vi "4155C Output v2.0.vi"(0 "VISA resource name in":refnum<visa-resource-name>="GPIB0::14::INSTR", 1 "Source/Common":u32(ring) items=["SMU1  ", "SMU2  ", "SMU3  ", "SMU4  ", "SMU5  ", "SMU6  "], 2 "Gate":T5={"Gate Start"=0.0, "Gate Stop"=0.0, "Gate Step"=0.0, "Gate Compliance"=0.1, "Gate PComp"=0.0, "Range mode"=0, "Range"=6} {"Range" max=11 scale=0.0..11.0; "Range mode" items=["Auto", "Limited", "Fixed"]; "Gate PComp" format="%^.2e"; "Gate Compliance" format="%^.2e"; "Gate Step" format="%^.4e"; "Gate Stop" format="%^.4e"; "Gate Start" format="%^.4e"}, 3 "Drain":T6={"Drain Start"=0.0, "Drain Stop"=0.0, "Drain Compliance"=0.1, "Drain Step (linear only)"=0.0, "Drain PComp"=0.0, "Range mode"=0, "Range"=6} {"Range" max=11 scale=0.0..11.0; "Range mode" items=["Auto", "Limited", "Fixed"]; "Drain PComp" format="%^.2e"; "Drain Step (linear only)" format="%^.4e"; "Drain Compliance" format="%^.2e"; "Drain Stop" format="%^.4e"; "Drain Start" format="%^.4e"}, 4 "Drain":u32(ring)=1 items=["SMU1  ", "SMU2  ", "SMU3  ", "SMU4  ", "SMU5  ", "SMU6  "], 5 "Timings":T4={"integration time"=0, "Short/Long integration time"=0.00064, "hold time (sec)"=0.0, "delay time (sec)"=0.0, "Step Time (0 disables)"=0.0, "sweep method"=0, "Pulse period"=0.005, "Base voltage"=0.0, "Pulse width"=0.0005} {"Pulse width" min=0.0005 max=0.1 step=0.0001 format="%.4f"; "Base voltage" format="%^.4e"; "Pulse period" min=0.005 max=1.0 step=0.0001 format="%.4f"; "sweep method" items=["Continuous", "Pulsed"]; "Step Time (0 disables)" format="%.2f"; "delay time (sec)" format="%.4f"; "hold time (sec)" format="%.4f"; "Short/Long integration time" format="%^.0e"; "integration time" scale=0.0..2.0}, 6 "error in (no error)":errorcluster, 7 "Probe 4":cluster{"on/off":bool, "Voltage":dbl} {"Voltage" min=-100.0 max=100.0 format="%.2f"}, 8 "Gate":u32(ring)=2 items=["SMU1  ", "SMU2  ", "SMU3  ", "SMU4  ", "SMU5  ", "SMU6  "], 9 "Probe 4":u32(ring)=3 items=["SMU1  ", "SMU2  ", "SMU3  ", "SMU4  ", "SMU5  ", "SMU6  "], 10 "sweep mode":u16(ring) items=["Single", "Double"], 12 "Panel controls":T3={"Emergency Stop"=refnum, "OutputGraph Max"=1e-05, "Text/Graph (text=false)"=FALSE} {"OutputGraph Max" format="%.2e"}, 13 "Standby":T1) -> (16 "VD":dbl[](array[numeric]) format="%.2f", 17 "Outparams":T2={"V2 Start"=0.0, "V2 Step"=0.0, "Number of points"=1} {"V2 Step" format="%.2f"; "V2 Start" format="%^.4e"}, 20 "VISA Resource Name out":refnum<visa-resource-name>, 22 "IS":dbl[](array[numeric]) format="%.2f", 23 "ID":dbl[](array[numeric]) format="%.2f", 25 "IG":dbl[](array[numeric]) format="%.2f", 26 "error out":errorcluster, 27 "Probe 4":dbl[](array[numeric]) format="%.2f")   [LabVIEW 2016]
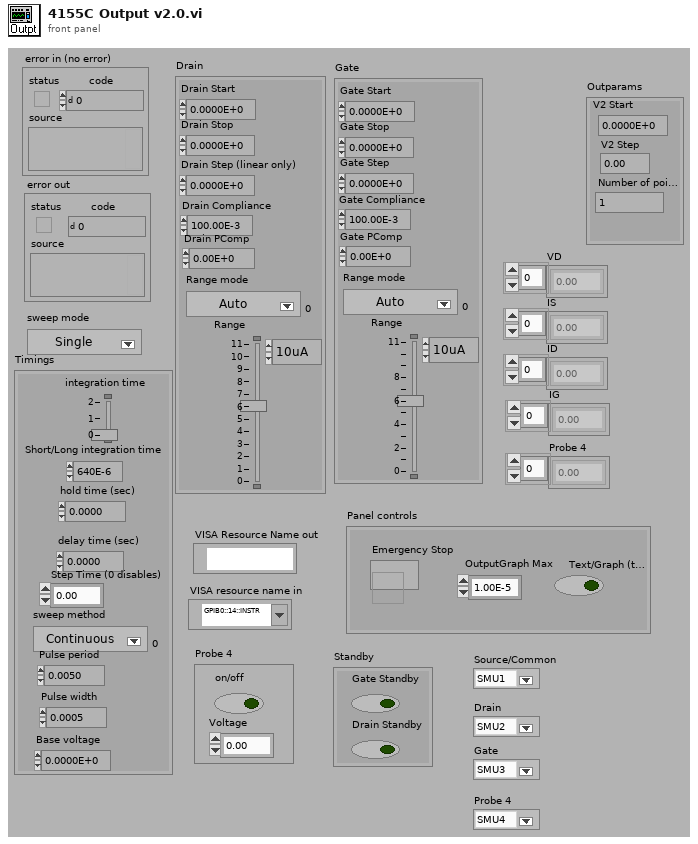
[diagram p1: front panel]
types:
  T1 = cluster{"Gate Standby":bool, "Drain Standby":bool}
  T2 = cluster{"V2 Start":dbl, "V2 Step":dbl, "Number of points":i32}
  T3 = cluster{"Emergency Stop":refnum<vi>, "OutputGraph Max":dbl, "Text/Graph (text=false)":bool}
  T4 = cluster{"integration time":u32, "Short/Long integration time":dbl, "hold time (sec)":dbl, "delay time (sec)":dbl, "Step Time (0 disables)":dbl, "sweep method":u16, "Pulse period":dbl, "Base voltage":dbl, "Pulse width":dbl}
  T5 = cluster{"Gate Start":dbl, "Gate Stop":dbl, "Gate Step":dbl, "Gate Compliance":dbl, "Gate PComp":dbl, "Range mode":u16, "Range":u8}
  T6 = cluster{"Drain Start":dbl, "Drain Stop":dbl, "Drain Compliance":dbl, "Drain Step (linear only)":dbl, "Drain PComp":dbl, "Range mode":u16, "Range":u8}
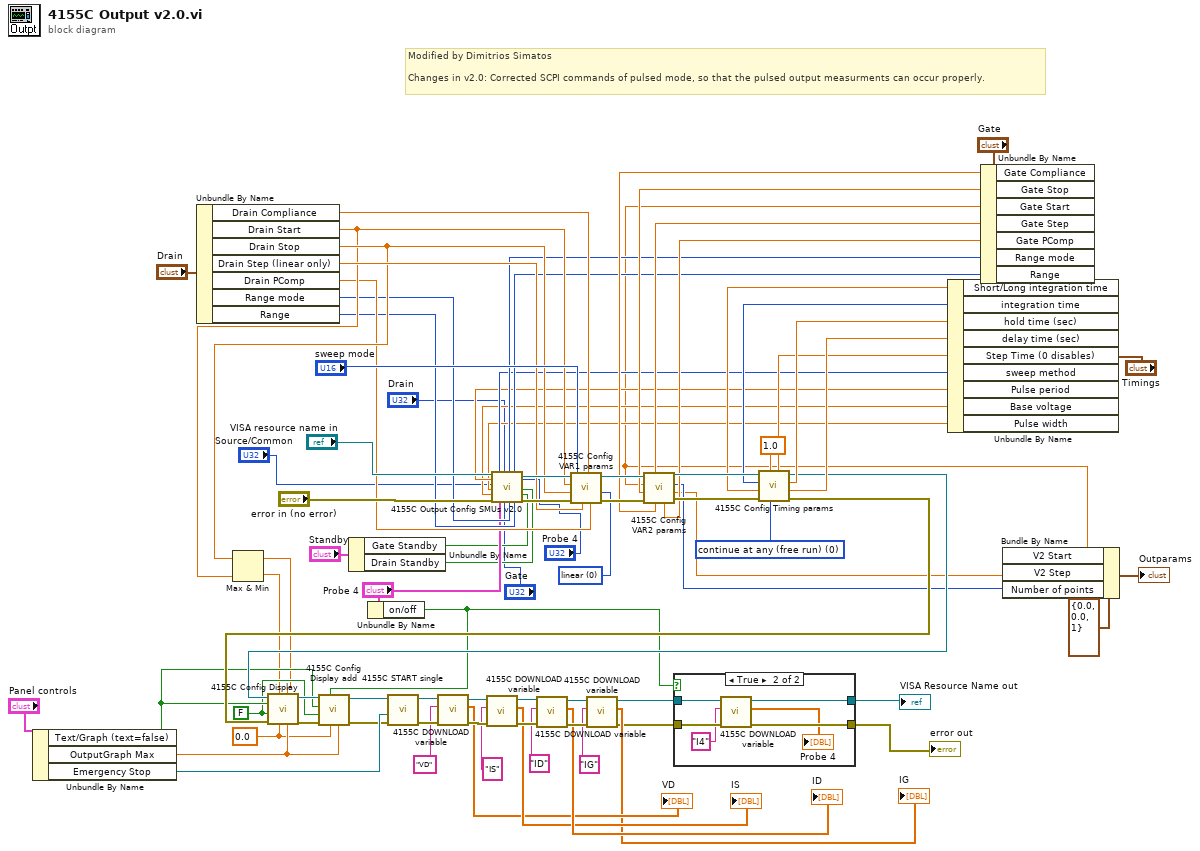
[diagram p0: block diagram]
diagram:
  w8 = 0.0 ("Ymin")
  w9 = FALSE ("Logarithmic")
  w69 = u8 0 items=["continue at any (free run)", "stop at any abnorm", "stop at compliance"] ("stop condition (free run:0)")
  w66 = u16 0 items=["linear", "log 10", "log 25", "log 50"] ("sweep spacing (linear: 0)")
  # "Modified by Dimitrios Simatos\n\nChanges in v2.0: Corrected SCPI commands of pulsed mode, so that the pulsed output measurments can occur properly."
  n1 = Unbundle By Name("Panel controls") -> ("Text/Graph (text=false)"=w10:bool, "OutputGraph Max"=w11:dbl, "Emergency Stop"=w39:refnum<vi>)
  n2 = Unbundle By Name("Drain") -> ("Drain Compliance"=w53:dbl, "Drain Start"=w41:dbl, "Drain Stop"=w42:dbl, "Drain Step (linear only)"=w52:dbl, "Drain PComp"=w38:dbl, "Range mode"=w34:u16, "Range"=w33:u8)
  n3 = Max & Min(x=w42, y=w41) -> (max(x,y)=w6:dbl, min(x,y)=w7:dbl)
  n4 = Unbundle By Name("Standby") -> ("Gate Standby"=w16:bool, "Drain Standby"=w17:bool)
  n5 = Unbundle By Name("Probe 4") -> ("on/off"=w5:bool)
  n6 = Unbundle By Name("Timings") -> ("Short/Long integration time"=w71:dbl, "integration time"=w48:u32, "hold time (sec)"=w49:dbl, "delay time (sec)"=w50:dbl, "Step Time (0 disables)"=w45:dbl, "sweep method"=w32:u16, "Pulse period"=w31:dbl, "Base voltage"=w29:dbl, "Pulse width"=w30:dbl)
  n7 = Unbundle By Name("Gate") -> ("Gate Compliance"=w56:dbl, "Gate Stop"=w55:dbl, "Gate Start"=w24:dbl, "Gate Step"=w54:dbl, "Gate PComp"=w37:dbl, "Range mode"=w36:u16, "Range"=w35:u8)
  n8 = call "4155C Output Config SMUs v2.0.vi"("VISA resource name in"="VISA resource name in", "Pulse period"=w31, "Source/Common"="Source/Common", "Pulse width"=w30, "Base voltage"=w29, "error in (no error)"="error in (no error)", "sweep method"=w32, "SMU4"="Probe 4", "Drain"="Drain", "Gate"="Gate", "Gate mode"=w36, "Source/drain mode"=w34, "Gate Range"=w35, "Source/drain Range"=w33, "Probe 4"="Probe 4", "Drain Standby"=w17, "Gate Standby"=w16) -> ("VISA Resource Name out"=w64:refnum<visa-resource-name>, "error out"=w63:errorcluster)  [unwired: 1 in]
  n9 = call "4155C Config VAR1 params.vi"("sweep spacing (linear: 0)"=w66, "power compliance (0 = OFF)"=w38, "compliance"=w53, "step (linear only)"=w52, "sweep mode"="sweep mode", "error in (no error)"=w63, "stop"=w42, "start"=w41, "VISA session"=w64) -> ("error out"=w67:errorcluster, "dup VISA resource name"=w68:refnum<visa-resource-name>)  [unwired: 1 out]
  n10 = call "4155C Config VAR2 params.vi"("power compliance (0 = OFF)"=w37, "compliance"=w56, "step"=w54, "error in (no error)"=w67, "stop"=w55, "start"=w24, "VISA session"=w68) -> ("error out"=w72:errorcluster, "Corrected Step"=w25:dbl, "Number of points"=w26:i32, "dup VISA resource name"=w73:refnum<visa-resource-name>)  [unwired: 1 in]
  n11 = call "4155C Config Timing params.vi"("delay time (sec)"=w50, "hold time (sec)"=w49, "Step Time (0 disables)"=w45, "stop condition (free run:0)"=w69, "wait time parameter"=1.0, "error in (no error)"=w72, "Short/Long integration time"=w71, "integration time"=w48, "VISA session"=w73) -> ("error out"=w44:errorcluster, "dup VISA resource name"=w43:refnum<visa-resource-name>)  [unwired: 1 in]
  n12 = call "4155C Config Display.vi"("Ymax"=w11, "Var1 Stop"=w6, "Ymin"=w8, "Var1 Start"=w7, "error in (no error)"=w44, "Logarithmic"=w9, "SPA Display"=w10, "VISA session"=w43) -> ("error out"=w12:errorcluster, "dup VISA resource name"=w15:refnum<visa-resource-name>)  [unwired: 2 in]
  n13 = call "4155C Config Display add.vi"("Ymax"=w11, "Ymin"=w8, "SMU4"=w5, "error in (no error)"=w12, "Logarithmic"=w9, "SPA Display"=w10, "VISA session"=w15) -> ("error out"=w13:errorcluster, "dup VISA resource name"=w14:refnum<visa-resource-name>)  [unwired: 3 in]
  n14 = call "4155C START single.vi"("error in (no error)"=w13, "Emergency Stop"=w39, "VISA resource name in"=w14) -> ("error out"=w84:errorcluster, "VISA Resource Name out"=w85:refnum<visa-resource-name>)  [unwired: 3 in]
  n15 = call "4155C DOWNLOAD variable.vi"("error in (no error)"=w84, "Variable name"="VD", "VISA resource name in"=w85) -> ("error out"=w82:errorcluster, "Output data"=→"VD":dbl[], "VISA Resource Name out"=w81:refnum<visa-resource-name>)  [unwired: 2 in]
  n16 = call "4155C DOWNLOAD variable.vi"("error in (no error)"=w82, "Variable name"="IS", "VISA resource name in"=w81) -> ("error out"=w78:errorcluster, "Output data"=→"IS":dbl[], "VISA Resource Name out"=w79:refnum<visa-resource-name>)  [unwired: 2 in]
  n17 = call "4155C DOWNLOAD variable.vi"("error in (no error)"=w78, "Variable name"="ID", "VISA resource name in"=w79) -> ("error out"=w77:errorcluster, "Output data"=→"ID":dbl[], "VISA Resource Name out"=w76:refnum<visa-resource-name>)  [unwired: 2 in]
  n18 = call "4155C DOWNLOAD variable.vi"("error in (no error)"=w77, "Variable name"="IG", "VISA resource name in"=w76) -> ("error out"=w19:errorcluster, "Output data"=→"IG":dbl[], "VISA Resource Name out"=w22:refnum<visa-resource-name>)  [unwired: 2 in]
  n19 = case shown="True" w5 {
    tunnel: w22 -> [w87 w93]
    tunnel: [w87 w90] -> w21
    tunnel: [w86 w91] -> w20
    tunnel: w19 -> [w86 w92]
    frame False {
    }
    frame True {
      n20 = call "4155C DOWNLOAD variable.vi"("error in (no error)"=w92, "Variable name"="I4", "VISA resource name in"=w93) -> ("error out"=w91:errorcluster, "Output data"=→"Probe 4":dbl[], "VISA Resource Name out"=w90:refnum<visa-resource-name>)  [unwired: 2 in]
    }
  }
  "error out" <- w20
  "VISA Resource Name out" <- w21
  n21 = Bundle By Name(cluster=T2 {"V2 Start"=0.0, "V2 Step"=0.0, "Number of points"=1} ("Outparams"), "V2 Start"=w24, "V2 Step"=w25, "Number of points"=w26) -> (→"Outparams":T2)
